vi "2005_FireAtSpecificMinutesEveryWednesday.vi"(8 "error in (no error)":errorcluster) -> (0 "error out":errorcluster)   [LabVIEW 2013]
uses:
  source/Cron.Jenkins/Cron.Jenkins.lvclass/Cron.Jenkins.ctl
  source/Cron.Jenkins/Write Job Name.vi
  <vilib>/addons/_JKI Toolkits/Caraya/classes/Assert/Assert True.vi
  source/Cron/Create Cron Expression.vi
  source/Cron/Compute Next Cron.vi
  source/Cron.Jenkins/Cron.Jenkins.lvclass
  <vilib>/addons/_JKI Toolkits/Caraya/classes/Test/Test.lvclass
  <vilib>/addons/_JKI Toolkits/Caraya/classes/Assert/Assert.lvclass
  source/openCron.lvlib
panel:
  out "after current month":timestamp
  out "Occurences":timestamp[](array[timestamp])
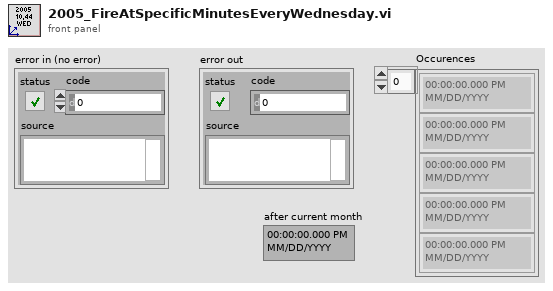
[diagram p1: front panel]
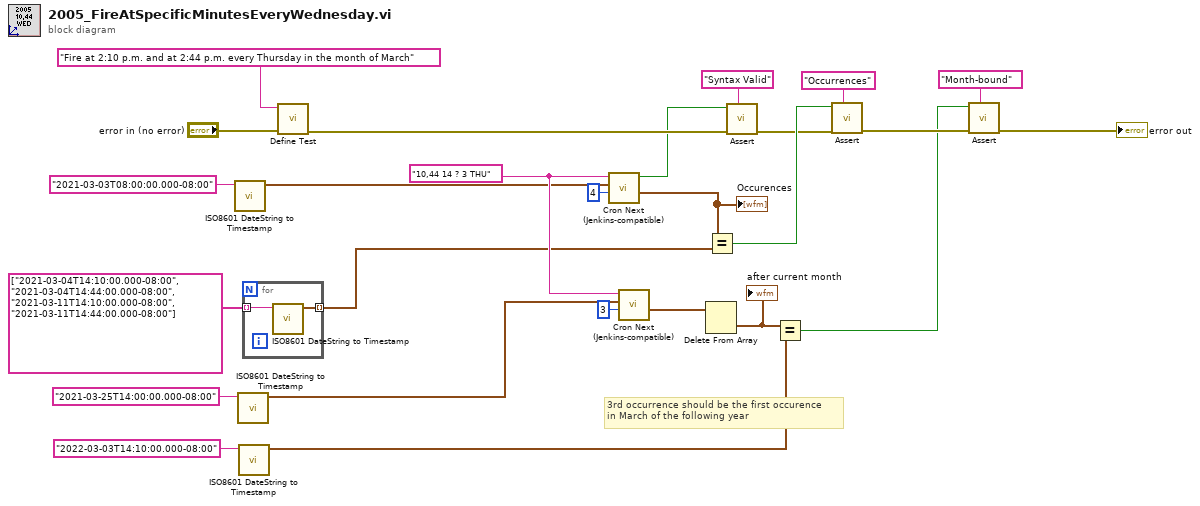
[diagram p0: block diagram]
diagram:
  w13 = "10,44 14 ? 3 THU" ("Expression")
  # "3rd occurrence should be the first occurence\nin March of the following year"
  n1 = call <vilib>:"ISO8601 DateString to Timestamp.vi"("ISO8601 Date String"="2021-03-03T08:00:00.000-08:00" ("Expression")) -> ("Timestamp"=w6:timestamp)  [unwired: 8 in, 2 out]
  n2 = call <vilib>:"ISO8601 DateString to Timestamp.vi"("ISO8601 Date String"="2021-03-25T14:00:00.000-08:00" ("Expression")) -> ("Timestamp"=w4:timestamp)  [unwired: 8 in, 2 out]
  n3 = call <vilib>:"ISO8601 DateString to Timestamp.vi"("ISO8601 Date String"="2022-03-03T14:10:00.000-08:00" ("Expression")) -> ("Timestamp"=w2:timestamp)  [unwired: 8 in, 2 out]
  n4 = for {
    tunnel: string[] ["2021-03-04T14:10:00.000-08:00", "2021-03-04T14:44:00.000-08:00", "2021-03-11T14:10:00.000-08:00", "2021-03-11T14:44:00.000-08:00"] -> [w28] mode=indexing
    tunnel: [w27] -> w1 mode=indexing
    n5 = call <vilib>:"ISO8601 DateString to Timestamp.vi"("ISO8601 Date String"=w28) -> ("Timestamp"=w27:timestamp)  [unwired: 8 in, 2 out]
  }
  n6 = call <vilib>:"Define Test.vi"("error in (no error)"="error in (no error)", "Label (VI Title)"="Fire at 2:10 p.m. and at 2:44 p.m. every Thursday in the month of March") -> ("error out"=w24:errorcluster)  [unwired: 8 in, 1 out]
  n7 = call "Cron Next (Jenkins-compatible).vi"("Nb Occurences (min: 1)"=u16 4, "Reference timestamp (Now)"=w6, "Cron Expression"=w13) -> ("Occurences"=w20:timestamp[], "syntax valid?"=w21:bool)  [unwired: 6 in, 1 out]
  "Occurences" <- w20
  n8 = call "Cron Next (Jenkins-compatible).vi"("Nb Occurences (min: 1)"=u16 3, "Reference timestamp (Now)"=w4, "Cron Expression"=w13) -> ("Occurences"=w10:timestamp[])  [unwired: 6 in, 2 out]
  n9 = Delete From Array(array=w10) -> (deleted portion=w9:timestamp)  [unwired: 2 in, 1 out]
  "after current month" <- w9
  n10 = Equal?(x=w20, y=w1) -> (x = y?=w23:bool)
  n11 = call-poly <vilib>:"Assert.vi"("Label"="Syntax Valid" ("Label (VI Title)"), "error in (no error)"=w24, "True?"=w21) -> ("error out"=w22:errorcluster)  [unwired: 7 in, 1 out]
  n12 = Equal?(x=w9, y=w2) -> (x = y?=w11:bool)
  n13 = call-poly <vilib>:"Assert.vi"("Label"="Occurrences" ("Label (VI Title)"), "error in (no error)"=w22, "True?"=w23) -> ("error out"=w15:errorcluster)  [unwired: 7 in, 1 out]
  n14 = call-poly <vilib>:"Assert.vi"("Label"="Month-bound" ("Label (VI Title)"), "error in (no error)"=w15, "True?"=w11) -> ("error out"=→"error out":errorcluster)  [unwired: 7 in, 1 out]
